vi "AD5933_ProgramFreqSweepParameter (NI-845x I2C)(SubVI).vi"(7 "error in":errorcluster, 9 "FrequencySweepConfigArray (Reg 0x82-0x8B)":T2, 10 "NI-845x Config for I2C (in)":cluster{"i2c configuration":T3, "Refnum in":T4}) -> (0 "error out":errorcluster, 3 "NI-845x Config for I2C (out)":T5)   [LabVIEW 2017]
uses:
  <vilib>/ni845x/ni845x.llb/ni845xI2cConfiguration.ctl
  <vilib>/ni845x/ni845x.llb/ni845xControl.ctl
  TypeDefs/AD5933_FreqSweepConfigRegisterArray.ctl
  TypeDefs/AD5933_CommandCodes.ctl
  TypeDefs/AD5933_Registers.ctl
panel:
  out "appended array":T1[](array[typedef]) format="%02x" items=["BlockWrite"=160, "BlockRead"=161, "AddressPointer"=176]
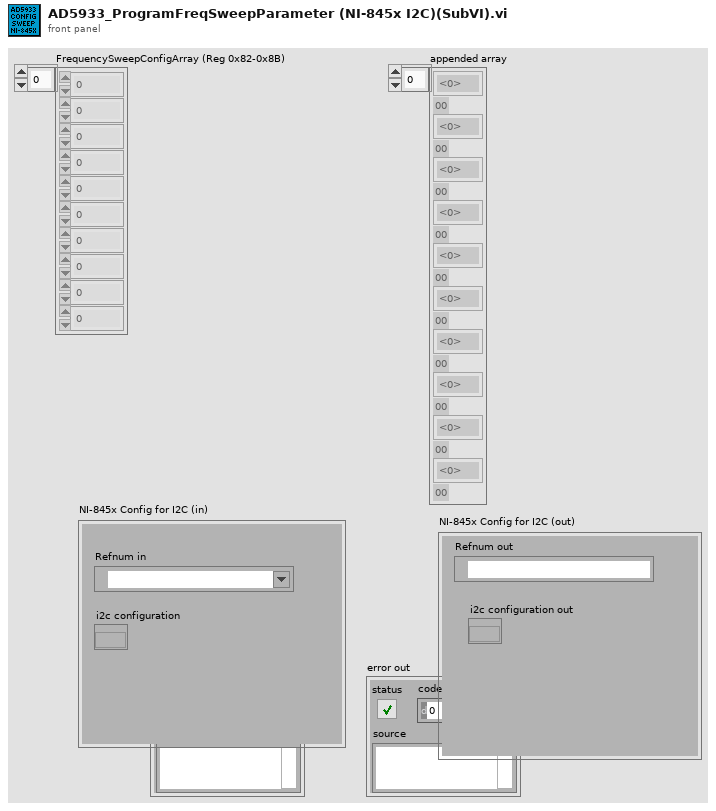
[diagram p1: front panel]
types:
  T1 = typedef "AD5933_CommandCodes.ctl" = u8
  T2 = typedef "AD5933_FreqSweepConfigRegisterArray.ctl" = u8[]
  T3 = typedef "ni845xI2cConfiguration.ctl" = refnum<k20>
  T4 = typedef "ni845xControl.ctl" = refnum<k21>
  T5 = cluster{"i2c configuration out":T3, "Refnum out":T4}
  T6 = typedef "AD5933_Registers.ctl" = u8
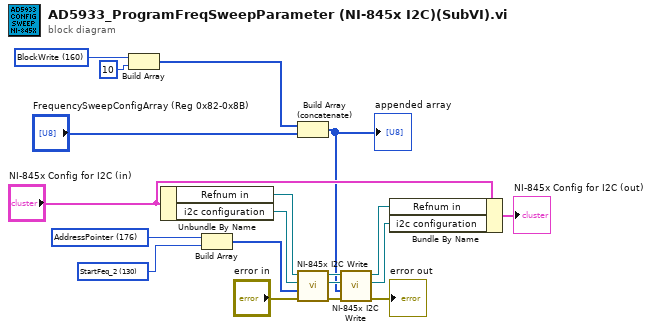
[diagram p0: block diagram]
diagram:
  w2 = T1 160 items=["BlockWrite"=160, "BlockRead"=161, "AddressPointer"=176] ("CommandCodes")
  w6 = T6 130 items=["Control_1"=128, "Control_0"=129, "StartFeq_2"=130, "StartFeq_1"=131, "StartFeq_0"=132, "FreqInc_2"=133, "FreqInc_1"=134, "FreqInc_0"=135, "NumOfInc_1"=136, "NumOfInc_0"=137, "NumOfSetCycl_1"=138, "NumOfSetCycl_0"=139, "Status"=143, "TempData_1"=146, "TempData_0"=147, "RealData_1"=148, "RealData_0"=149, "ImagData_1"=150, "ImagData_0"=151] ("Register")
  w7 = T1 176 items=["BlockWrite"=160, "BlockRead"=161, "AddressPointer"=176] ("CommandCodes")
  n1 = Build Array(w2, 10) -> (w5:i32[])
  n2 = Unbundle By Name("NI-845x Config for I2C (in)") -> ("Refnum in"=w11:T4, "i2c configuration"=w12:T3)
  n3 = Build Array(w7, w6) -> (w19:T6[])
  n4 = Build Array (concatenate)(w5, "FrequencySweepConfigArray (Reg 0x82-0x8B)") -> (w3:i32[])
  "appended array" <- w3
  n5 = call <vilib>:"NI-845x I2C Write.vi"("error in (no error)"="error in", "write data"=w19, "i2c configuration in"=w12, "device reference in"=w11) -> ("error out"=w18:errorcluster, "i2c configuration out"=w16:T3, "device reference out"=w15:T4)  [unwired: 5 in]
  n6 = call <vilib>:"NI-845x I2C Write.vi"("error in (no error)"=w18, "write data"=w3, "i2c configuration in"=w16, "device reference in"=w15) -> ("error out"=→"error out":errorcluster, "i2c configuration out"=w9:T3, "device reference out"=w10:T4)  [unwired: 5 in]
  n7 = Bundle By Name(cluster="NI-845x Config for I2C (in)", "Refnum in"=w10, "i2c configuration"=w9) -> (→"NI-845x Config for I2C (out)":cluster{"i2c configuration":T3, "Refnum in":T4})
